vi "Update Value & Color.vi"(0 "Ref In":refnum<vi>, 1 "Thresold Array & Range Max":dbl[](array[numeric]), 2 "BG Color In":u32, 3 "Ref type In":T1(ring), 4 "Control Label In":string, 5 "Calculated Value (F)?":bool, 6 "Val Change?":bool, 7 "Value In":sgl[](array[numeric])) -> (14 "Ref type":T1(ring), 15 "BG Color":u32)   [LabVIEW 2018]
uses:
  <vilib>/ptbypt/NI_PtbyPt.lvlib
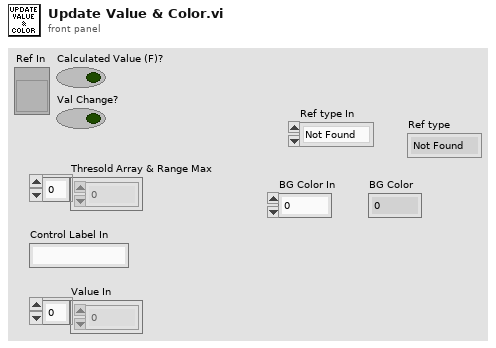
[diagram p1: front panel]
types:
  T1 = enum16{"Not Found", "Knob", "Numeric", "Slide", "String", "Boolean"}
  T2 = enum16{"Not Found", "Knob", "Numeric", "Slide", "String", "Boolean"}[]
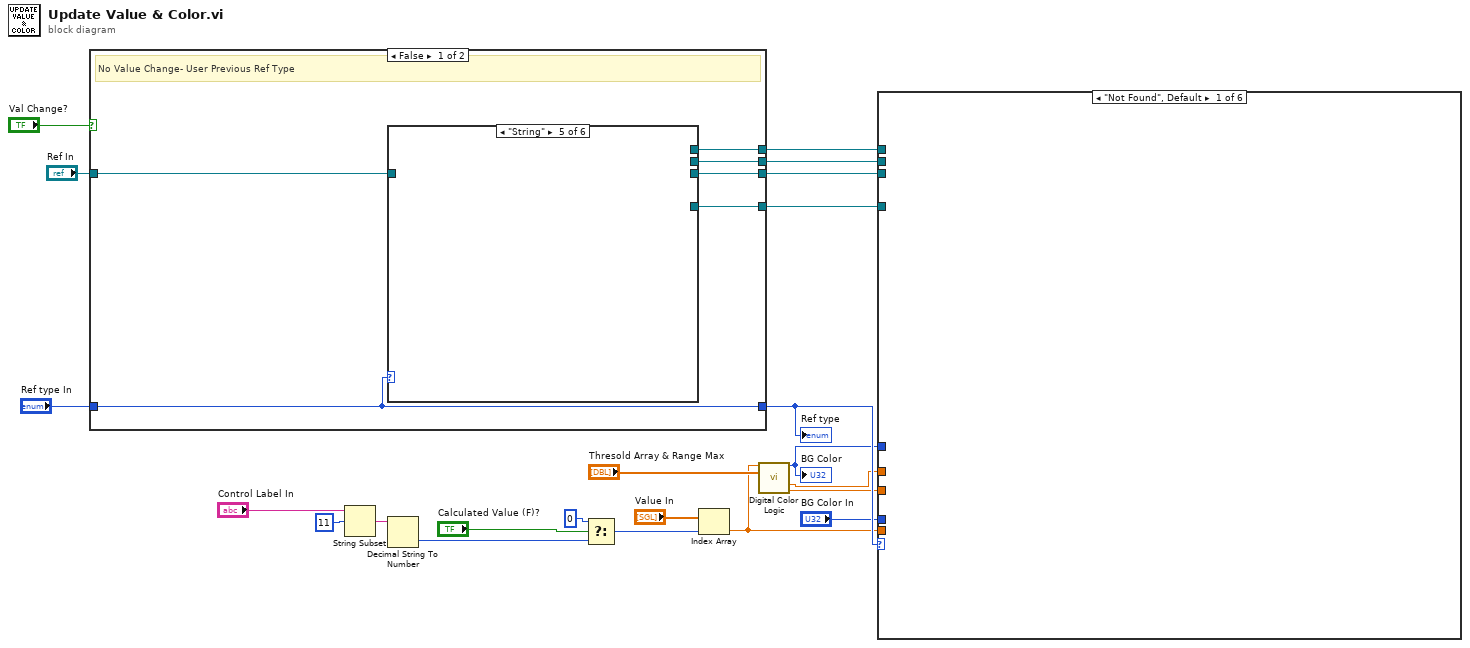
[diagram p0: block diagram]
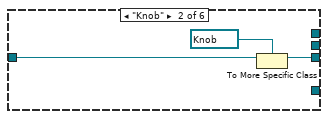
[diagram p3: hidden frame]
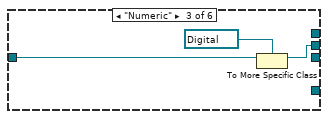
[diagram p4: hidden frame]
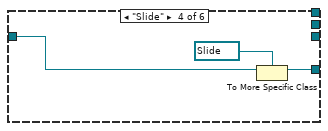
[diagram p5: hidden frame]
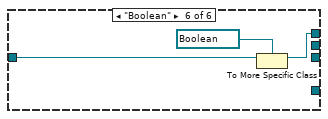
[diagram p6: hidden frame]
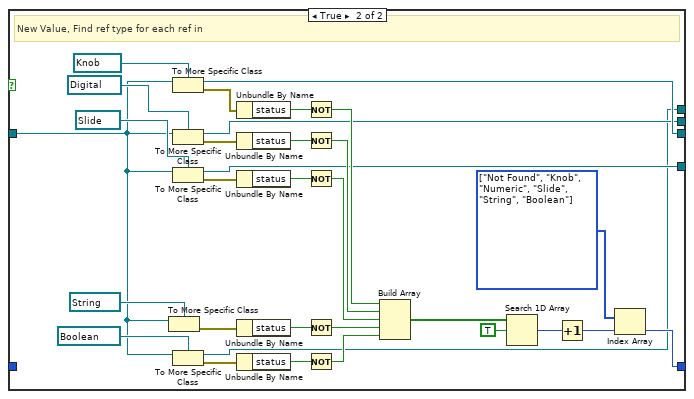
[diagram p7: hidden frame]
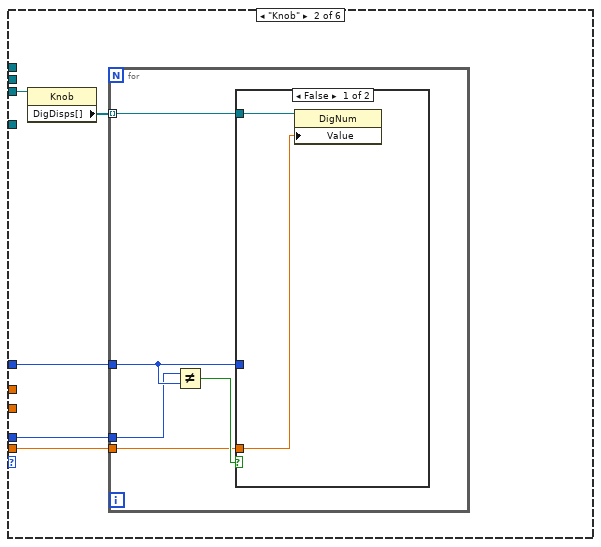
[diagram p8: hidden frame]
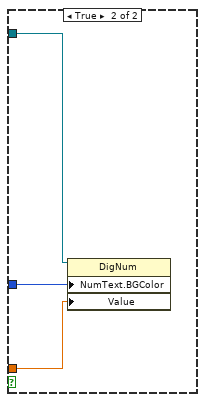
[diagram p9: hidden frame]
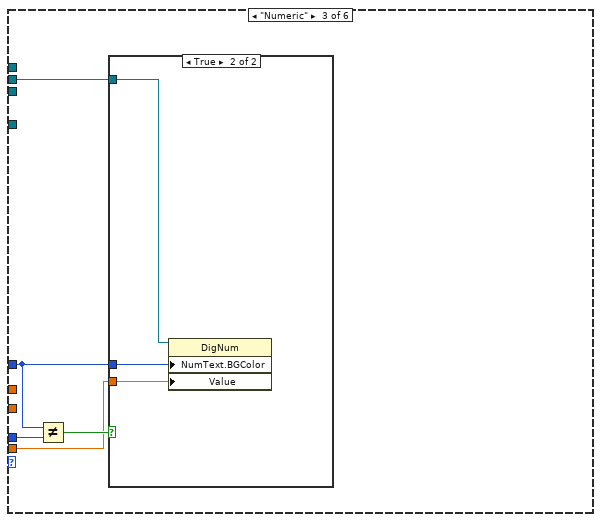
[diagram p10: hidden frame]
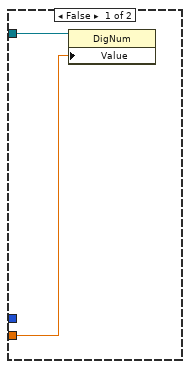
[diagram p11: hidden frame]
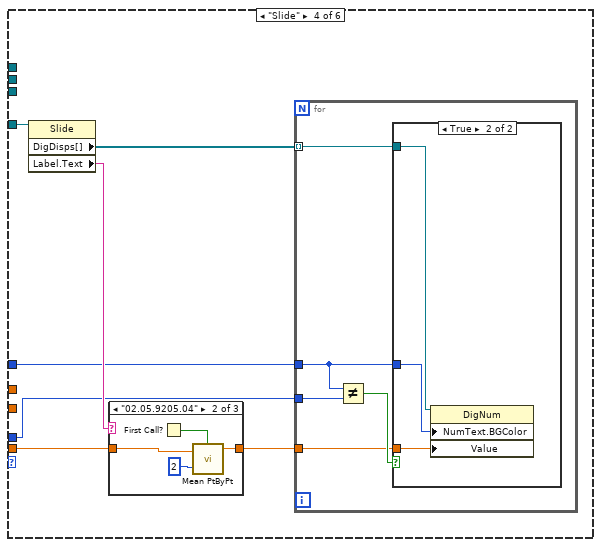
[diagram p12: hidden frame]
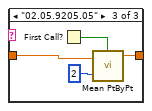
[diagram p14: hidden frame]
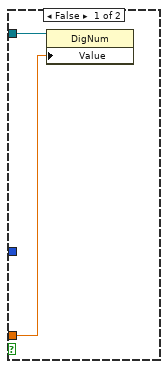
[diagram p15: hidden frame]
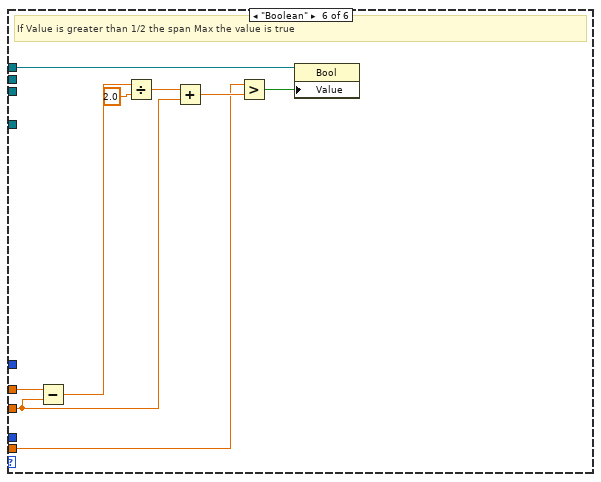
[diagram p17: hidden frame]
diagram:
  n1 = case shown="False" "Val Change?" {
    tunnel: [w23 w46] -> w17
    tunnel: [w27 w45] -> w15
    tunnel: [w25 w44] -> w14
    tunnel: [w26 w43] -> w13
    tunnel: [w24 w42] -> w12
    tunnel: "Ref type In" -> [w23 _]
    tunnel: "Ref In" -> [w28 w41]
    frame False {
      # "No Value Change- User Previous Ref Type"
      n2 = case shown="\"String\"" w23 {
        tunnel: [_ _ w34 _ _ _] -> w26
        tunnel: w28 -> [_ w30 w32 w36 _ w39]
        tunnel: [_ w29 _ _ _ _] -> w27
        tunnel: [_ _ _ w35 _ _] -> w25
        tunnel: [_ _ _ _ _ w38] -> w24
        frame "Not Found", Default {
        }
        frame "Knob" {
          n3 = To More Specific Class(target class=refnum<vi> refnum ("Control Ref"), reference=w30) -> (specific class reference=w29:refnum<vi>)  [unwired: 1 in, 1 out]
        }
        frame "Numeric" {
          n4 = To More Specific Class(target class=refnum<vi> refnum ("Control Ref"), reference=w32) -> (specific class reference=w34:refnum<vi>)  [unwired: 1 in, 1 out]
        }
        frame "Slide" {
          n5 = To More Specific Class(target class=refnum<vi> refnum ("Control Ref"), reference=w36) -> (specific class reference=w35:refnum<vi>)  [unwired: 1 in, 1 out]
        }
        frame "String" {
        }
        frame "Boolean" {
          n6 = To More Specific Class(target class=refnum<vi> refnum ("Control Ref"), reference=w39) -> (specific class reference=w38:refnum<vi>)  [unwired: 1 in, 1 out]
        }
      }
    }
    frame True {
      w52 = T2 [enum."Not Found", enum."Knob", enum."Numeric", enum."Slide", enum."String", enum."Boolean"] items=["Not Found", "Knob", "Numeric", "Slide", "String", "Boolean"]
      # "New Value, Find ref type for each ref in"
      n7 = To More Specific Class(target class=refnum<vi> refnum ("Control Ref"), reference=w41) -> (error out=w62:errorcluster)  [unwired: 1 in, 1 out]
      n8 = To More Specific Class(target class=refnum<vi> refnum ("Control Ref"), reference=w41) -> (specific class reference=w45:refnum<vi>, error out=w71:errorcluster)  [unwired: 1 in]
      n9 = To More Specific Class(target class=refnum<vi> refnum ("Control Ref"), reference=w41) -> (specific class reference=w43:refnum<vi>, error out=w63:errorcluster)  [unwired: 1 in]
      n10 = To More Specific Class(target class=refnum<vi> refnum ("Control Ref"), reference=w41) -> (specific class reference=w44:refnum<vi>, error out=w64:errorcluster)  [unwired: 1 in]
      n11 = To More Specific Class(target class=refnum<vi> refnum ("Control Ref"), reference=w41) -> (specific class reference=w42:refnum<vi>, error out=w48:errorcluster)  [unwired: 1 in]
      n12 = Unbundle By Name(w71) -> ("status"=w70:bool)
      n13 = Unbundle By Name(w63) -> ("status"=w66:bool)
      n14 = Unbundle By Name(w64) -> ("status"=w65:bool)
      n15 = Unbundle By Name(w62) -> ("status"=w61:bool)
      n16 = Unbundle By Name(w48) -> ("status"=w49:bool)
      n17 = Not(x=w70) -> (.not. x?=w59:bool)
      n18 = Not(x=w66) -> (.not. x?=w58:bool)
      n19 = Not(x=w65) -> (.not. x?=w57:bool)
      n20 = Not(x=w61) -> (.not. x?=w56:bool)
      n21 = Not(x=w49) -> (.not. x?=w47:bool)
      n22 = Build Array(w59, w58, w57, w56, w47) -> (w55:bool[])
      n23 = Search 1D Array(1D array=w55, element=TRUE) -> (index of element=w53:i32)  [unwired: 1 in]
      n24 = Increment(x=w53) -> (x+1=w51:i32)
      n25 = Index Array(array=w52, index=w51) -> (element=w46:T1)
    }
  }
  "Ref type" <- w17
  n26 = String Subset(string="Control Label In", offset (0)=11) -> (substring=w20:string)  [unwired: 1 in]
  n27 = Decimal String To Number(string=w20) -> (number=w9:i32)  [unwired: 2 in, 1 out]
  n28 = Select(t=0, s="Calculated Value (F)?", f=w9) -> (s? t:f=w7:i32)
  n29 = Index Array(array="Value In", index=w7) -> (element=w16:sgl)
  n30 = call "Digital Color Logic.vi"("Sensor Value"=w16, "Thresold Array"="Thresold Array & Range Max") -> ("Color Out"=w1:u32, "Span Max"=w11:dbl, "Span Min"=w10:dbl)  [unwired: 9 in, 2 out]
  "BG Color" <- w1
  n31 = case shown="\"Not Found\", Default" w17 {
    tunnel: w16 -> [_ w73 w88 w100 _ w125]
    tunnel: w1 -> [_ w75 w90 w98 _ _]
    tunnel: w15 -> [_ w74 _ _ _ _]
    tunnel: w14 -> [_ _ _ w103 _ _]
    tunnel: w13 -> [_ _ w89 _ _ _]
    tunnel: w12 -> [_ _ _ _ _ w130]
    tunnel: w11 -> [_ _ _ _ _ w124]
    tunnel: w10 -> [_ _ _ _ _ w123]
    tunnel: "BG Color In" -> [_ w72 w87 w97 _ _]
    frame "Not Found", Default {
    }
    frame "Knob" {
      n32 = property class="Knob"(reference=w74) -> ("DigDisps[]"=w76:refnum<vi>[])  [unwired: 1 in, 2 out]
      n33 = for {
        tunnel: w73 -> [w78]
        tunnel: w76 -> [w79] mode=indexing
        tunnel: w75 -> [w80]
        tunnel: w72 -> [w77]
        n34 = Not Equal?(x=w77, y=w80) -> (x != y?=w81:bool)
        n35 = case shown="False" w81 {
          tunnel: w79 -> [w83 w86]
          tunnel: w80 -> [_ w85]
          tunnel: w78 -> [w82 w84]
          frame False {
            n36 = property class="DigNum"(reference=w83, "Value"=w82) -> ()  [unwired: 1 in, 2 out]
          }
          frame True {
            n37 = property class="DigNum"(reference=w86, "NumText.BGColor"=w85, "Value"=w84) -> ()  [unwired: 1 in, 2 out]
          }
        }
      }
    }
    frame "Numeric" {
      n38 = Not Equal?(x=w90, y=w87) -> (x != y?=w91:bool)
      n39 = case shown="True" w91 {
        tunnel: w89 -> [w92 w96]
        tunnel: w90 -> [_ w95]
        tunnel: w88 -> [w93 w94]
        frame False {
          n40 = property class="DigNum"(reference=w92, "Value"=w93) -> ()  [unwired: 1 in, 2 out]
        }
        frame True {
          n41 = property class="DigNum"(reference=w96, "NumText.BGColor"=w95, "Value"=w94) -> ()  [unwired: 1 in, 2 out]
        }
      }
    }
    frame "Slide" {
      n42 = property class="Slide"(reference=w103) -> ("DigDisps[]"=w102:refnum<vi>[], "Label.Text"=w101:string)  [unwired: 1 in, 2 out]
      n43 = case shown="\"02.05.9205.04\"" w101 {
        tunnel: w100 -> [w104 w108 w112]
        tunnel: [w104 w107 w111] -> w99
        frame Default {
        }
        frame "02.05.9205.04" {
          n44 = First Call?() -> (First Call?: T/F=w106:bool)
          n45 = call <vilib>:"Mean PtByPt.vi"("x"=w108, "sample length"=2, "initialize"=w106) -> ("mean"=w107:dbl)  [unwired: 1 in, 1 out]
        }
        frame "02.05.9205.05" {
          n46 = First Call?() -> (First Call?: T/F=w110:bool)
          n47 = call <vilib>:"Mean PtByPt.vi"("x"=w112, "sample length"=2, "initialize"=w110) -> ("mean"=w111:dbl)  [unwired: 1 in, 1 out]
        }
      }
      n48 = for {
        tunnel: w99 -> [w114]
        tunnel: w102 -> [w115] mode=indexing
        tunnel: w98 -> [w116]
        tunnel: w97 -> [w113]
        n49 = Not Equal?(x=w116, y=w113) -> (x != y?=w117:bool)
        n50 = case shown="True" w117 {
          tunnel: w115 -> [w118 w122]
          tunnel: w116 -> [_ w121]
          tunnel: w114 -> [w119 w120]
          frame False {
            n51 = property class="DigNum"(reference=w118, "Value"=w119) -> ()  [unwired: 1 in, 2 out]
          }
          frame True {
            n52 = property class="DigNum"(reference=w122, "NumText.BGColor"=w121, "Value"=w120) -> ()  [unwired: 1 in, 2 out]
          }
        }
      }
    }
    frame "String" {
      # "No Need for String Ref"
    }
    frame "Boolean" {
      # "If Value is greater than 1/2 the span Max the value is true"
      n53 = Subtract(x=w124, y=w123) -> (x-y=w128:dbl)
      n54 = Divide(x=w128, y=2.0) -> (x/y=w127:dbl)
      n55 = Add(x=w127, y=w123) -> (x+y=w126:dbl)
      n56 = Greater?(x=w125, y=w126) -> (0:w131:bool)
      n57 = property class="Bool"(reference=w130, "Value"=w131) -> ()  [unwired: 1 in, 2 out]
    }
  }
